vi "LV_GetVSLogs_TS_Step.vi"(0 "Engine Reference":refnum<k7>, 1 "Condition Run?":bool, 2 "First call":bool, 5 "Sequence File Ref":refnum<k7>, 7 "Logs Folder":string="\"C:\\\\Users\\\\Public\\\\Documents\\\\National Instruments\\\\VeriStand\\\\Logs\\\\NIGEL\"", 11 "error in":errorcluster, 13 "index":i32, 14 "Sequence Name":string="MainSequence") -> (3 "First call out":bool, 4 "Engine reference(out)":refnum<k7>, 6 "Sequence File Ref(out)":refnum<k7>, 15 "error out":errorcluster)   [LabVIEW 2011]
doc: "This VI creates a TestStand step that calls a LabVIEW VI that gets the latest file created in the selected folder (Logs Folder) and stores the file path in a TS local variable"
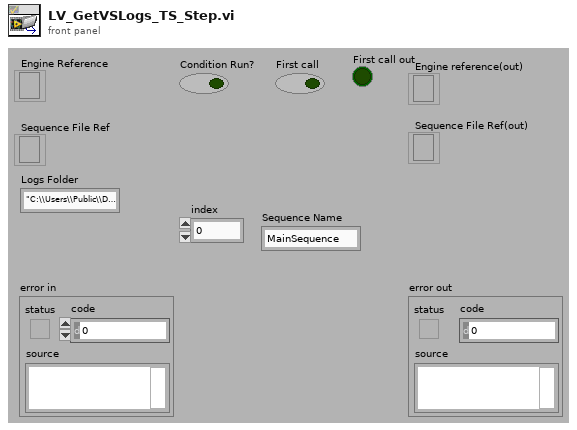
[diagram p1: front panel]
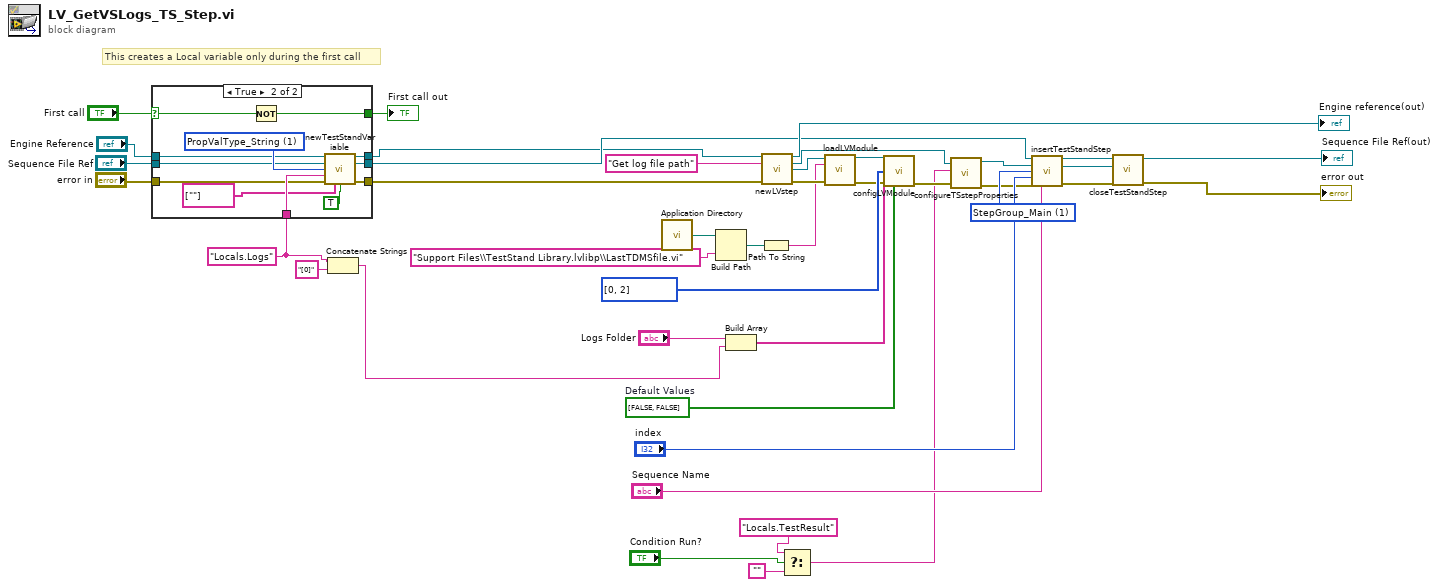
[diagram p0: block diagram]
diagram:
  w11 = "Locals.Logs" ("Variable Name")
  w25 = bool[] [FALSE, FALSE]  # Default Values
  w34 = 1 items=["StepGroup_Setup", "StepGroup_Main", "StepGroup_Cleanup"] ("Step Group")
  # "This creates a Local variable only during the first call"
  n1 = case shown="True" "First call" {
    selector: "First call" -> [w45 w52]
    tunnel: [w44 w57] -> w3
    tunnel: [w43 w56] -> w7
    tunnel: w11 -> [_ w54]
    tunnel: [w42 w53] -> w8
    tunnel: [w45 w51] -> w9
    tunnel: "Sequence File Ref" -> [w43 w50]
    tunnel: "error in" -> [w42 w49]
    tunnel: "Engine Reference" -> [w44 w48]
    frame False {
    }
    frame True {
      w55 = 1 items=["PropValType_Container", "PropValType_String", "PropValType_Boolean", "PropValType_Number", "PropValType_NamedType", "PropValType_Reference", "PropValType_Array"] ("Variable Type")
      n2 = Not(x=w52) -> (.not. x?=w51:bool)
      n3 = call "newTestStandVariable.vi"("Engine Reference"=w48, "Sequence File Ref"=w50, "Variable Type"=w55, "Variable Name"=w54, "error in"=w49, "Variable Value"=string[] [""], "Array?"=TRUE) -> ("Engine Reference(out)"=w57:refnum<k7>, "Sequence File Ref(out)"=w56:refnum<k7>, "error out"=w53:errorcluster)  [unwired: 6 in]
    }
  }
  "First call out" <- w9
  n4 = Concatenate Strings(w11, "[0]" ("string")) -> (w2:string)
  n5 = call <vilib>:"Application Directory.vi"() -> ("Application Directory"=w1:path)
  n6 = Build Path(base path=w1, name or relative path="Support Files\\TestStand Library.lvlibp\\LastTDMSfile.vi") -> (appended path=w22:path)
  n7 = Build Array("Logs Folder", w2) -> (w26:string[])
  n8 = Path To String(path=w22) -> (string=w21:string)
  n9 = call "newLVstep.vi"("Engine Reference"=w3, "Step Name"="Get log file path", "error in"=w8) -> ("Engine reference(out)"=→"Engine reference(out)":refnum<k7>, "NewStep (out)"=w17:refnum<k7>, "LV Module (out)"=w37:refnum<k7>, "error out"=w36:errorcluster)  [unwired: 9 in]
  n10 = Select(t="Locals.TestResult", s="Condition Run?", f="") -> (s? t:f=w13:string)
  n11 = call "loadLVModule.vi"("LV Module"=w37, "VIPath"=w21, "error in"=w36) -> ("LV Module(out)"=w38:refnum<k7>, "error out"=w39:errorcluster)  [unwired: 11 in]
  n12 = call "configLVModule.vi"("LV Module"=w38, "Parameter Indices"=i32[] [0, 2], "Param values"=w26, "error in"=w39, "Default Values"=w25) -> ("error out"=w20:errorcluster)  [unwired: 10 in]
  n13 = call "configureTSstepProperties.vi"("error in"=w20, "Precondition"=w13, "NewStep (in)"=w17) -> ("error out"=w19:errorcluster, "NewStep (out)"=w18:refnum<k7>)  [unwired: 7 in]
  n14 = call "insertTestStandStep.vi"("Sequence File Ref"=w7, "Step to insert"=w18, "Step Group"=w34, "index"="index", "error out"=w19, "Sequence Name"="Sequence Name") -> ("Sequence File Ref(out)"=w29:refnum<k7>, "Step to insert (out)"=w30:refnum<k7>, "error out"=w35:errorcluster)  [unwired: 7 in]
  n15 = call "closeTestStandStep.vi"("error in"=w35, "NewStep"=w30, "Sequence File Ref"=w29) -> ("error out"=→"error out":errorcluster, "Sequence File Ref(out)"=→"Sequence File Ref(out)":refnum<k7>)  [unwired: 7 in]
